vi "Get 3.5 char times.vi"(7 "wait multiplier":sgl=1.0, 11 "baud rate":u32) -> (3 "wait time (ms)":u32, 5 "initial wait (ms)":u32)   [LabVIEW 2013, in "Modbus Library - Advance.lvlib" / "Serial Shared Components.lvlib"]
uses:
  Serial Shared Components.lvlib
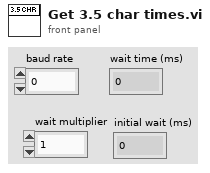
[diagram p1: front panel]
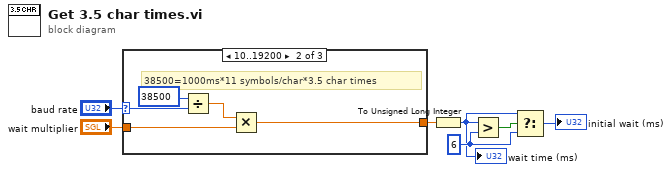
[diagram p0: block diagram]
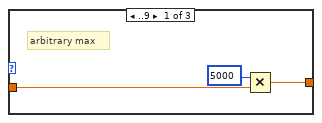
[diagram p2: hidden frame]
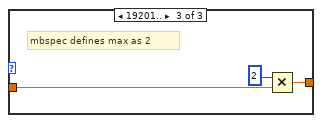
[diagram p3: hidden frame]
diagram:
  w4 = u32 6 ("y")
  n1 = case shown="10..19200" "baud rate" {
    selector: "baud rate" -> [_ w14 _]
    tunnel: [w9 w11 w17] -> w5
    tunnel: "wait multiplier" -> [w8 w12 w16]
    frame ..9 {
      # "arbitrary max"
      n2 = Multiply(x=u32 5000, y=w8) -> (x*y=w9:sgl)
    }
    frame 10..19200 {
      # "38500=1000ms*11 symbols/char*3.5 char times"
      n3 = Divide(x=u32 38500 ("y"), y=w14) -> (x/y=w15:dbl)
      n4 = Multiply(x=w15, y=w12) -> (x*y=w11:dbl)
    }
    frame 19201.. {
      # "mbspec defines max as 2"
      n5 = Multiply(x=u32 2, y=w16) -> (x*y=w17:sgl)
    }
  }
  n6 = To Unsigned Long Integer(number=w5) -> (unsigned 32bit integer=w1:u32)
  "wait time (ms)" <- w1
  n7 = Greater?(x=w1, y=w4) -> (0:w6:bool)
  n8 = Select(t=w1, s=w6, f=w4) -> (s? t:f=→"initial wait (ms)":u32)
